vi "SaveToDataFile.vi"(8 "error in":errorcluster, 10 "Readout in":dbl[][](array[numeric]), 11 "File Paths":T1={"Local Save Path"=path "\\\\smbhome.uscs.susx.ac.uk\\cv222/Desktop/data", "Newton Save Path"=path "Z:/#Projects/Entanglement/data", "File Name"="test", "LocalSave"=TRUE}) -> (0 "error out":errorcluster, 3 "New data?":bool=TRUE)   [LabVIEW 2017]
uses:
  controls/FilePaths.ctl
  controls/GlobalExp.vi
  <vilib>/Utility/file.llb/Write To Spreadsheet File (string).vi
  <vilib>/Utility/file.llb/Write To Spreadsheet File (DBL).vi
  Global.lvlib
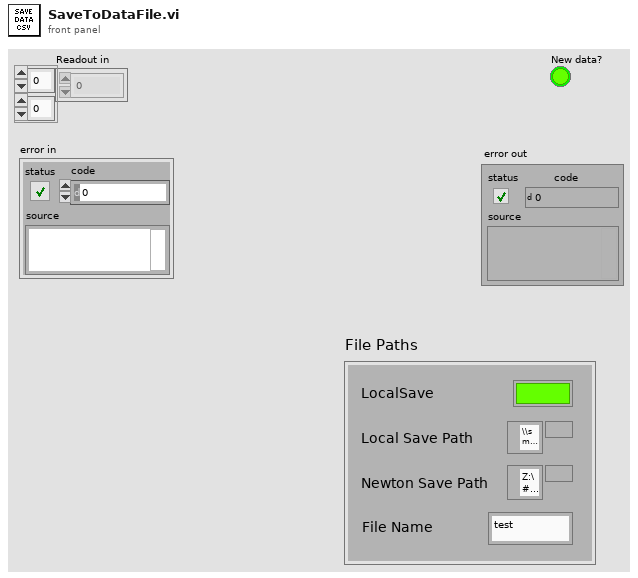
[diagram p1: front panel]
types:
  T1 = typedef "FilePaths.ctl" = cluster{"Local Save Path":path, "Newton Save Path":path, "File Name":string, "LocalSave":bool}
  T2 = typedef "MasterExpControl.ctl" = cluster{"Main Steps":dbl, "Main Runs":dbl, "ExpStatus":enum16{"Innit", "Stop", "Idle", "MainRunning", "AuxRunning"}, "Main Current Step":dbl, "ExpNum":dbl, "NewData":bool, "date":string, "command":string, "Stop":bool, "Pause":bool, "Mathematica":string, "Main/Meta":bool, "UpdateMath":bool, "Camera":bool}
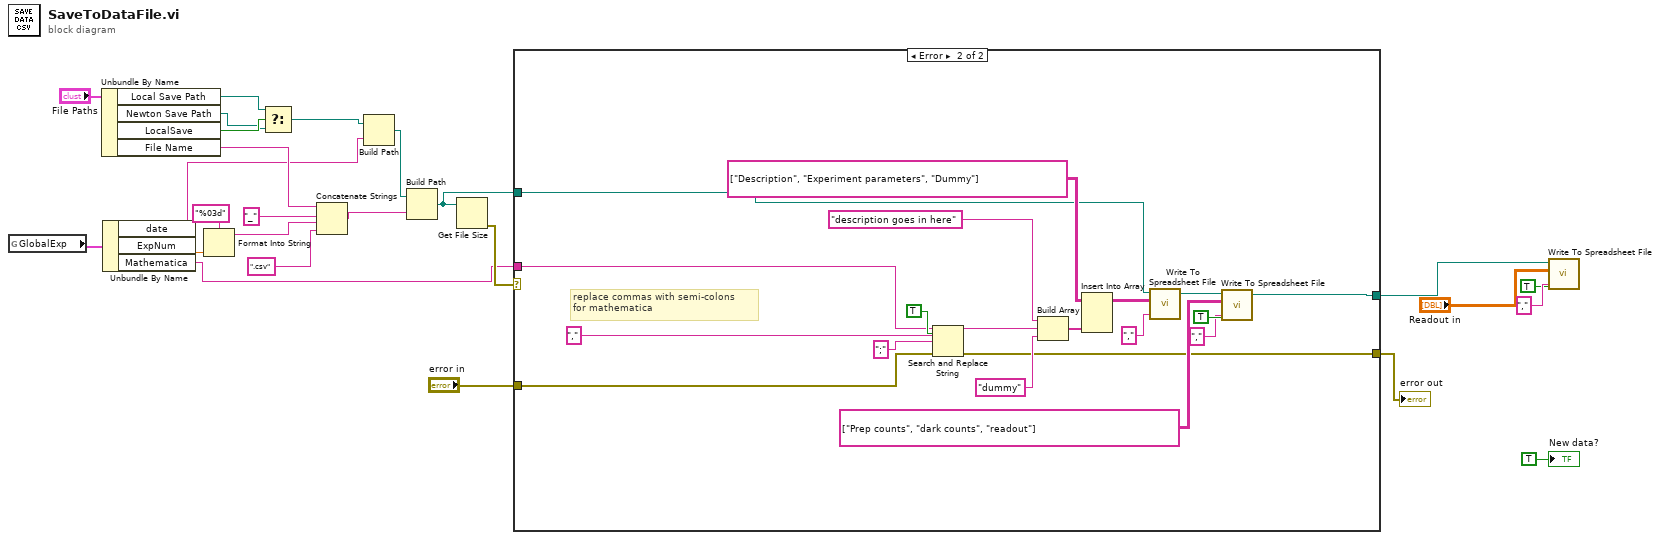
[diagram p0: block diagram]
diagram:
  n1 = global read "GlobalExp.vi" "GlobalExp"() -> (w21:T2)
  n2 = Unbundle By Name("File Paths") -> ("Local Save Path"=w22:path, "Newton Save Path"=w23:path, "LocalSave"=w24:bool, "File Name"=w20:string)
  n3 = Unbundle By Name(w21) -> ("date"=w13:string, "ExpNum"=w11:dbl, "Mathematica"=w4:string)
  n4 = Format Into String(format string="%03d", w11) -> (resulting string=w16:string)  [unwired: 2 in, 1 out]
  n5 = Select(t=w22, s=w24, f=w23) -> (s? t:f=w14:path)
  n6 = Concatenate Strings(w20, "_", w16, ".csv") -> (w18:string)
  n7 = Build Path(base path=w14, name or relative path=w13) -> (appended path=w12:path)
  n8 = Build Path(base path=w12, name or relative path=w18) -> (appended path=w9:path)
  n9 = Get File Size(file=w9) -> (0:w10:errorcluster)  [unwired: 1 in, 2 out]
  n10 = case shown="Error" w10 {
    tunnel: w9 -> [w27 w32]
    tunnel: [w27 w31] -> w5
    tunnel: w4 -> [_ w30]
    tunnel: [w26 w29] -> w2
    tunnel: "error in" -> [w26 w28]
    frame No Error {
    }
    frame Error {
      # "replace commas with semi-colons \nfor mathematica"
      n11 = Search and Replace String(replace all?=TRUE ("replace all? (F)"), input string=w30, search string=",", replace string=";" ("replace string (\"\")"), error in=w28) -> (result string=w36:string, error out=w29:errorcluster)  [unwired: 3 in, 2 out]
      n12 = Build Array("description goes in here" ("element"), w36, "dummy" ("element")) -> (w40:string[])
      n13 = Insert Into Array(array=string[][] [["Description", "Experiment parameters", "Dummy"]], new element=w40) -> (w41:string[][])  [unwired: 2 in]
      n14 = call-poly <vilib>:"Write To Spreadsheet File.vi"("delimiter (\\t)"="," ("delimiter (\\t)"), "2D data"=w41, "file path (dialog if empty)"=w32) -> ("new file path (Not A Path if cancelled)"=w45:path)  [unwired: 5 in]
      n15 = call-poly <vilib>:"Write To Spreadsheet File.vi"("delimiter (\\t)"="," ("delimiter (\\t)"), "append to file? (new file:F)"=TRUE, "2D data"=string[][] [["Prep counts", "dark counts", "readout"]], "file path (dialog if empty)"=w45) -> ("new file path (Not A Path if cancelled)"=w31:path)  [unwired: 4 in]
    }
  }
  "error out" <- w2
  n16 = call-poly <vilib>:"Write To Spreadsheet File.vi"("delimiter (\\t)"="," ("delimiter (\\t)"), "append to file? (new file:F)"=TRUE, "2D data"="Readout in", "file path (dialog if empty)"=w5) -> ()  [unwired: 4 in, 1 out]
  "New data?" <- TRUE ("Boolean")
